vi "Release Singleton.vi"(8 "error in (no error)":errorcluster, 11 "PrefsDB in":refnum<class "PrefsDB.lvclass">) -> (0 "error out":errorcluster)   [LabVIEW 2020, in "User Prefs.lvlib" / "PrefsDB.lvclass"]
uses:
  PrefsDB.lvclass
  PrefsDB.lvclass/PrefsDB.ctl
  lv-cdm/CDM-Config/Config Manager/Config Manager.lvclass
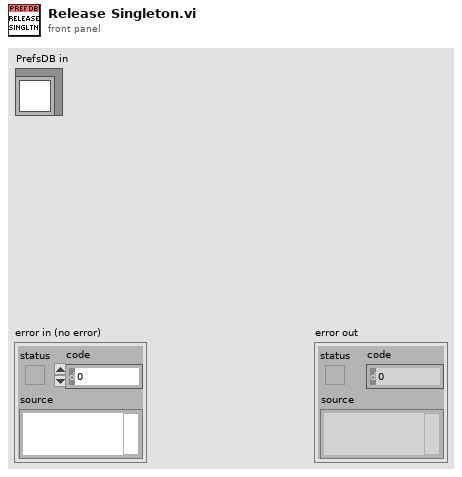
[diagram p1: front panel]
types:
  T1 = typedef "User Prefs.lvlib/PrefsDB.lvclass/Ref Data.ctl" = cluster{"Map":map{string, T2}}
  T2 = typedef "User Prefs.lvlib/PrefsDB.lvclass/Pref Group.ctl" = cluster{"Config Manager":refnum<class "Config Manager.lvclass">, "Group":string}
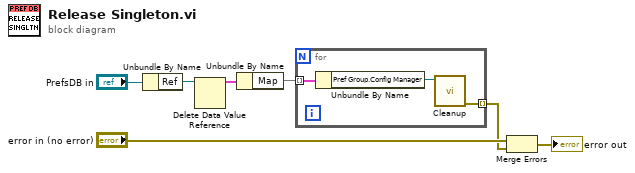
[diagram p0: block diagram]
diagram:
  n1 = Unbundle By Name("PrefsDB in") -> ("Ref"=w5:refnum<data-value>)
  n2 = Delete Data Value Reference(data value reference=w5) -> (data value=w4:T1)  [unwired: 1 in, 1 out]
  n3 = Unbundle By Name(w4) -> ("Map"=w3:map{string, T2})
  n4 = for {
    tunnel: w3 -> [w10] mode=indexing
    tunnel: [w8] -> w1 mode=indexing
    n5 = Unbundle By Name(w10) -> ("Pref Group.Config Manager"=w9:refnum<class "Config Manager.lvclass">)
    n6 = call "Cleanup.vi"("Config Manager in"=w9) -> ("error out"=w8:errorcluster)  [unwired: 10 in]
  }
  n7 = Merge Errors("error in (no error)", w1) -> (→"error out":errorcluster)
